vi "Test Suite Disable Methods.vi"(8 "error in (no error)":errorcluster, 11 "Test Case In":refnum<class "LUnit Test Suite Tests.lvclass">) -> (0 "error out":errorcluster, 3 "Test Case Out":refnum<class "LUnit Test Suite Tests.lvclass">)   [LabVIEW 2020, in "LUnit Test Suite Tests.lvclass"]
uses:
  LUnit Test Suite Tests.lvclass
  C:/Program Files (x86)/National Instruments/LabVIEW 2020/vi.lib/Astemes/LUnit/Test Case.lvclass
  LUnit Test Case Tests/LUnit Test Case V2 Test Double/LUnit Test Case V2 Test Double.lvclass
  C:/Git/astemes-lunit/source/Rewrite Project/LUnit Test Case/LUnit Test Case V2.lvclass
  <vilib>/Astemes/LUnit/Test Case.lvclass/Test Case.ctl
  b74e4934-f044-4222-b3dd-fc90e6c1bd4f.vi
  <vilib>/Astemes/LUnit/Palette/Pass.vi
  <vilib>/Astemes/LUnit/Palette/Fail.vi
  <vilib>/Astemes/LUnit/Compare Variants.vi
  <vilib>/Astemes/LUnit/Describe Comparison.vi
  <vilib>/Astemes/LUnit/Set Assertion Type.vi
  <vilib>/Astemes/LUnit/Add test result.vi
  <vilib>/Astemes/LUnit/Variant to string.vi
  <vilib>/Astemes/LUnit/LUnit Record Assertion Result.vi
  <vilib>/Astemes/LUnit/LUnit Aggregate Assertion Results.vi
  <vilib>/Astemes/LUnit/Method Result/LUnit Merge Status.vi
  <vilib>/Astemes/LUnit/LUnit Concatenate result strings.vi
  <vilib>/Utility/Data Type/Get Type Information.vi
  <vilib>/Utility/LVClass/Get LV Class Name.vi
  LUnit Test Suite/LUnit Test Suite V2.lvclass
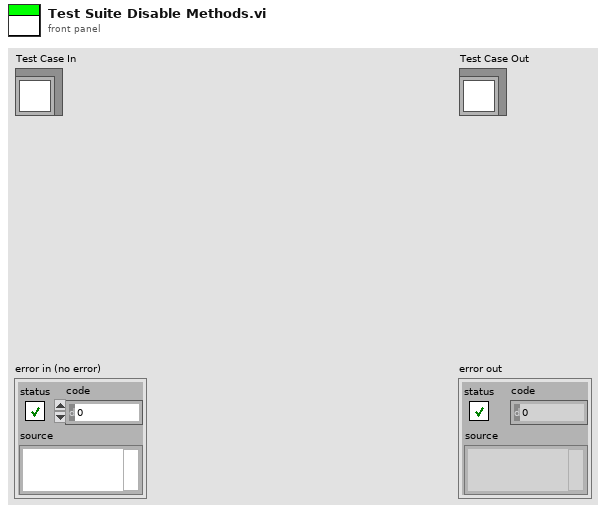
[diagram p1: front panel]
types:
  T1 = typedef "Result.lvlib/Result.ctl" = cluster{"Case":string, "Method":string, "Message":string, "Description":string, "Status":T2, "Result Type":T3, "Execution Time":dbl}
  T2 = typedef "Result.lvlib/Status.ctl" = enum16{"Pass", "Fail", "Error", "Skipped", "Setup Error", "Broken", "Teardown Error"}
  T3 = typedef "Result.lvlib/Type.ctl" = enum16{"Assertion", "Method", "Case", "Suite"}
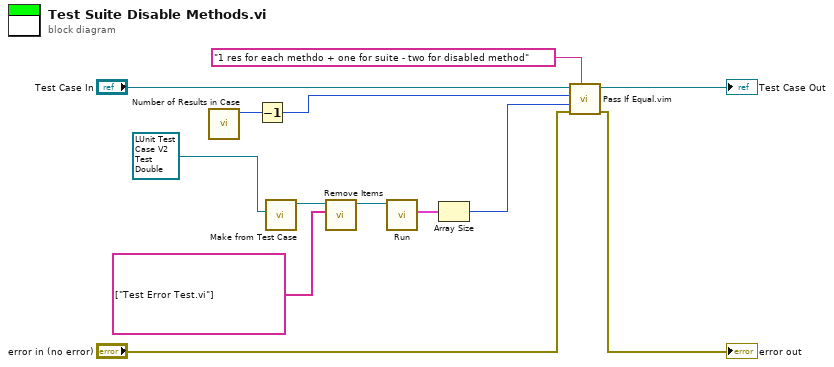
[diagram p0: block diagram]
diagram:
  n1 = call "Number of Results in Case.vi"() -> ("Number of Results"=w6:i32)  [unwired: 11 in]
  n2 = Decrement(x=w6) -> (x-1=w1:i32)
  n3 = call "Make from Test Case.vi"("LUnit Test Case"=refnum<class "LUnit Test Case V2 Test Double.lvclass"> refnum ("LUnit Test Case V2 Test Double.lvclass")) -> ("LUnit Test Suite V2 out"=w8:refnum<class "LUnit Test Suite V2.lvclass">)  [unwired: 9 in, 1 out]
  n4 = call "Remove Items.vi"("Methods"=string[] ["Test Error Test.vi"], "LUnit Test Suite V2 in"=w8) -> ("LUnit Test Suite V2 out"=w4:refnum<class "LUnit Test Suite V2.lvclass">)  [unwired: 8 in, 1 out]
  n5 = call-dynamic "Run.vi"("Run in"=w4) -> ("Results"=w9:T1[])  [unwired: 9 in, 1 out]
  n6 = Array Size(array=w9) -> (size(s)=w5:i32)
  n7 = call "Pass If Equal.vim"("Description"="1 res for each methdo + one for suite - two for disabled method", "error in (no error)"="error in (no error)", "Actual"=w5, "Expected"=w1, "LUnit Test Case In"="Test Case In") -> ("error out"=→"error out":errorcluster, "LUnit Test Case Out"=→"Test Case Out":refnum<class "LUnit Test Suite Tests.lvclass">)  [unwired: 5 in]
